vi "BotSpeak_Waitms.vi"(2 "Wait (ms)":dbl=1.0, 3 "Bot Settings":T1) -> (1 "Bot Settings 2":T1)   [LabVIEW 2014]
doc: "Causes VI to wait the specified number of milliseconds."
uses:
  <userlib>/BotSpeak/VIs/Direct/BotSpeak_Control.ctl
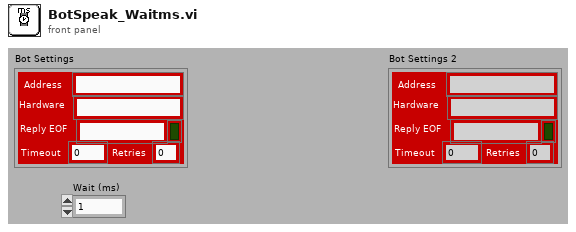
[diagram p1: front panel]
types:
  T1 = typedef "BotSpeak_Control.ctl" = cluster{"Address":string, "Reply EOF":string, "Hardware":string, "Retries":i8, "Timeout":i32, "Open?":bool}
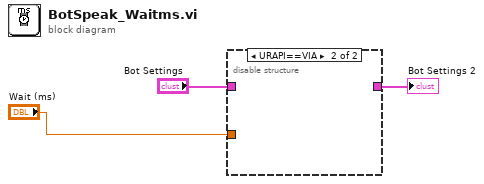
[diagram p0: block diagram]
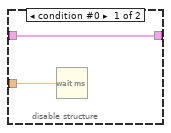
[diagram p2: hidden frame]
diagram:
  n1 = disable-structure shown="URAPI==VIA" {
    disable-tunnel: "Wait (ms)" -> [w5 _]
    disable-tunnel: "Bot Settings" -> [w4 _]
    disable-tunnel: [w4 _] -> w1
    frame condition #0 {
      n2 = Wait (ms)(milliseconds to wait=w5) -> ()  [unwired: 1 out]
    }
    frame condition #1 (active) {
    }
  }
  "Bot Settings 2" <- w1
